vi "Rotate2DArray.vi"(9 "Direction (clockwise)":T1(ring), 11 "Array in":dbl[][](array[numeric])) -> (3 "Array Out":dbl[][](array[numeric]))   [LabVIEW 2014]
doc: "This VI demonstrates how to rotate a 2D-array 90 degrees clockwise or counter-clockwise using array transposition and row reverse operations."
panel:
  # "1. Choose the Direction to rotate the 2D-array\n2. Run the VI\n\nFor further information, choose Help > Show Context Help\nand hover the mouse over the icon above."
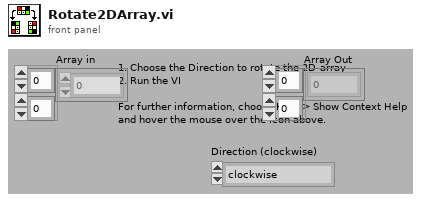
[diagram p1: front panel]
types:
  T1 = enum16{"clockwise", "counter-clockwise", "nothing"}
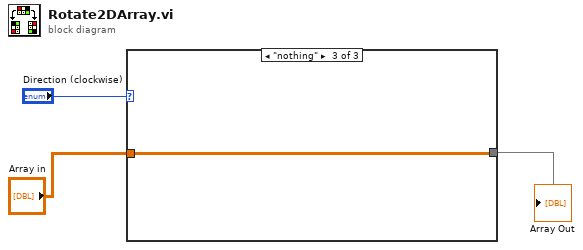
[diagram p0: block diagram]
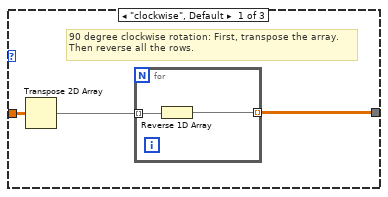
[diagram p2: hidden frame]
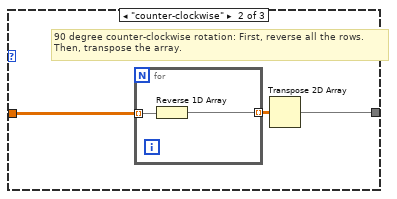
[diagram p3: hidden frame]
diagram:
  n1 = case shown="\"nothing\"" "Direction (clockwise)" {
    tunnel: "Array in" -> [w6 w9 w14]
    tunnel: [w4 w10 w14] -> w2
    frame "clockwise", Default {
      # "90 degree clockwise rotation: First, transpose the array.\nThen reverse all the rows."
      n2 = Transpose 2D Array(2D array=w6) -> (transposed array=w5:dbl[][])
      n3 = for {
        tunnel: w5 -> [w8] mode=indexing
        tunnel: [w7] -> w4 mode=indexing
        n4 = Reverse 1D Array(array=w8) -> (reversed array=w7:dbl[])
      }
    }
    frame "counter-clockwise" {
      # "90 degree counter-clockwise rotation: First, reverse all the rows.\nThen, transpose the array."
      n5 = for {
        tunnel: w9 -> [w13] mode=indexing
        tunnel: [w12] -> w11 mode=indexing
        n6 = Reverse 1D Array(array=w13) -> (reversed array=w12:dbl[])
      }
      n7 = Transpose 2D Array(2D array=w11) -> (transposed array=w10:dbl[][])
    }
    frame "nothing" {
    }
  }
  "Array Out" <- w2
